vi "Get Sibling.vi"(8 "error in (no error)":errorcluster, 11 "NodeRef In":refnum<data-value>) -> (0 "error out":errorcluster, 2 "Sibling":refnum<data-value>, 3 "NodeRef":refnum<data-value>)   [LabVIEW 2020]
uses:
  Node.lvclass
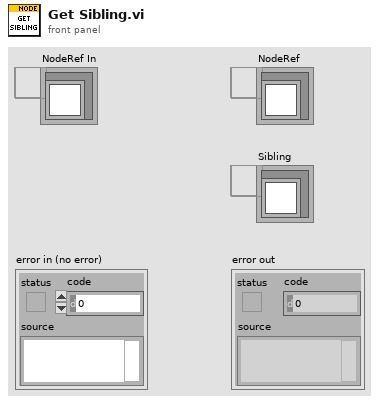
[diagram p1: front panel]
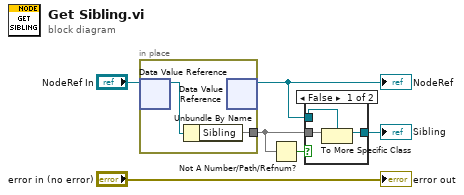
[diagram p0: block diagram]
diagram:
  n1 = in-place {
    in-place-border: [w7] -> w3
    n2 = in-place-dvr #1("NodeRef In") -> (w8:refnum<class "Node.lvclass">)  [unwired: 1 out]
    n3 = Unbundle By Name(w8) -> ("Sibling"=w7)
    n4 = in-place-dvr #1() -> (w2:refnum<data-value>)  [unwired: 1 in, 1 out]
  }
  "NodeRef" <- w2
  n5 = Not A Number/Path/Refnum?(number/path/refnum=w3) -> (NaN/Path/Refnum?=w4:bool)
  n6 = case shown="False" w4 {
    tunnel: w3 -> [w11 _]
    tunnel: w2 -> [w10 _]
    tunnel: [w9 _] -> w1
    frame False {
      n7 = To More Specific Class(target class=w10, reference=w11) -> (specific class reference=w9:refnum<data-value>)  [unwired: 1 in, 1 out]
    }
    frame True {
    }
  }
  "Sibling" <- w1
  "error out" <- "error in (no error)"
